vi "Process_Oculus_Data - Rufus.vi"(5 "Arm X Min":dbl, 7 "Arm X Max":dbl, 8 "error in":errorcluster, 9 "Calibration Data in":T3, 10 "Calibrated":bool, 11 "Raw Oculus Data":T1) -> (0 "error out":errorcluster, 1 "Calibration Data out":T3, 3 "Calibrated Oculus Data":T2)   [LabVIEW 2017]
uses:
  Calibrated Oculus Data.ctl
  Raw Oculus Data.ctl
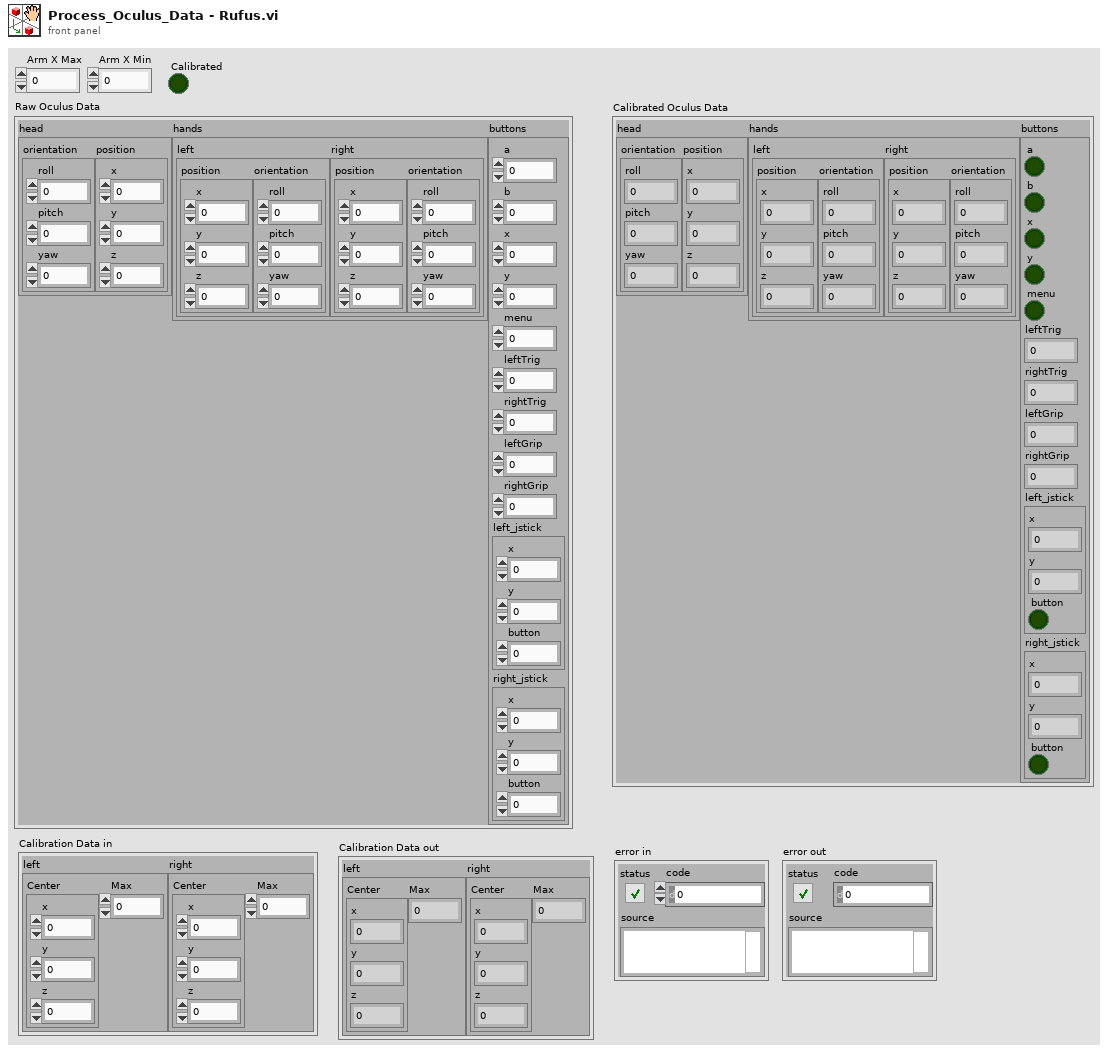
[diagram p1: front panel]
types:
  T1 = typedef "Raw Oculus Data.ctl" = cluster{"head":cluster{"orientation":cluster{"roll":dbl, "pitch":dbl, "yaw":dbl}, "position":cluster{"x":dbl, "y":dbl, "z":dbl}}, "hands":cluster{"left":cluster{"position":cluster{"x":dbl, "y":dbl, "z":dbl}, "orientation":cluster{"roll":dbl, "pitch":dbl, "yaw":dbl}}, "right":cluster{"position":cluster{"x":dbl, "y":dbl, "z":dbl}, "orientation":cluster{"roll":dbl, "pitch":dbl, "yaw":dbl}}}, "buttons":cluster{"a":i32, "b":i32, "x":i32, "y":i32, "menu":i32, "leftTrig":dbl, "rightTrig":dbl, "leftGrip":dbl, "rightGrip":dbl, "left_jstick":cluster{"x":dbl, "y":dbl, "button":i32}, "right_jstick":cluster{"x":dbl, "y":dbl, "button":i32}}}
  T2 = typedef "Calibrated Oculus Data.ctl" = cluster{"head":cluster{"orientation":cluster{"roll":dbl, "pitch":dbl, "yaw":dbl}, "position":cluster{"x":dbl, "y":dbl, "z":dbl}}, "hands":cluster{"left":cluster{"position":cluster{"x":dbl, "y":dbl, "z":dbl}, "orientation":cluster{"roll":dbl, "pitch":dbl, "yaw":dbl}}, "right":cluster{"position":cluster{"x":dbl, "y":dbl, "z":dbl}, "orientation":cluster{"roll":dbl, "pitch":dbl, "yaw":dbl}}}, "buttons":cluster{"a":bool, "b":bool, "x":bool, "y":bool, "menu":bool, "leftTrig":dbl, "rightTrig":dbl, "leftGrip":dbl, "rightGrip":dbl, "left_jstick":cluster{"x":dbl, "y":dbl, "button":bool}, "right_jstick":cluster{"x":dbl, "y":dbl, "button":bool}}}
  T3 = cluster{"left":cluster{"Center":cluster{"x":dbl, "y":dbl, "z":dbl}, "Max":dbl}, "right":cluster{"Center":cluster{"x":dbl, "y":dbl, "z":dbl}, "Max":dbl}}
  T4 = typedef "Calibration Control.ctl" = enum16{"Calibrate", "Max", "Min"}
  T5 = cluster{"orientation":cluster{"roll":dbl, "pitch":dbl, "yaw":dbl}, "position":cluster{"x":dbl, "y":dbl, "z":dbl}}
  T6 = cluster{"left":cluster{"position":cluster{"x":dbl, "y":dbl, "z":dbl}, "orientation":cluster{"roll":dbl, "pitch":dbl, "yaw":dbl}}, "right":cluster{"position":cluster{"x":dbl, "y":dbl, "z":dbl}, "orientation":cluster{"roll":dbl, "pitch":dbl, "yaw":dbl}}}
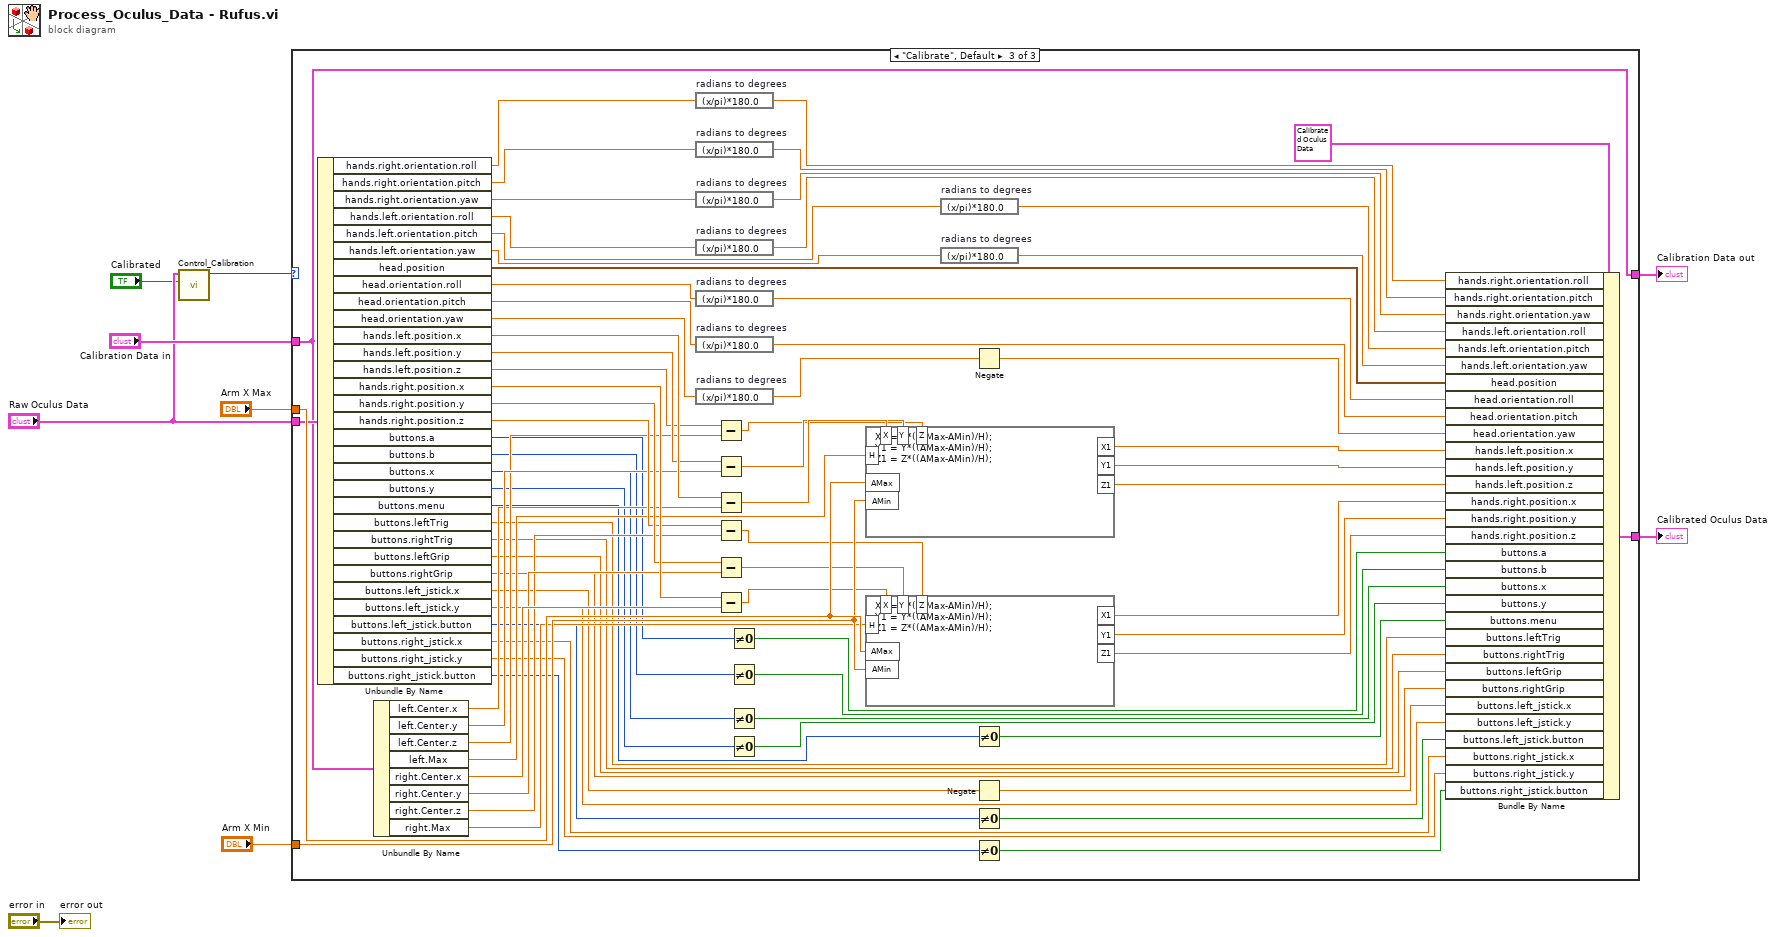
[diagram p0: block diagram]
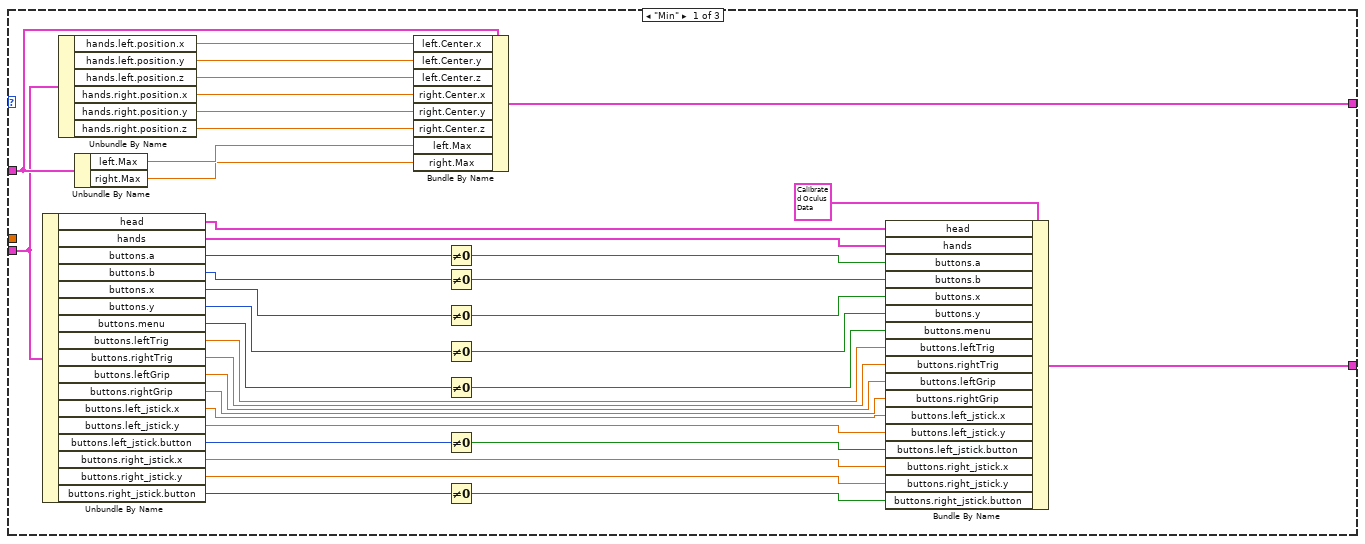
[diagram p2: hidden frame]
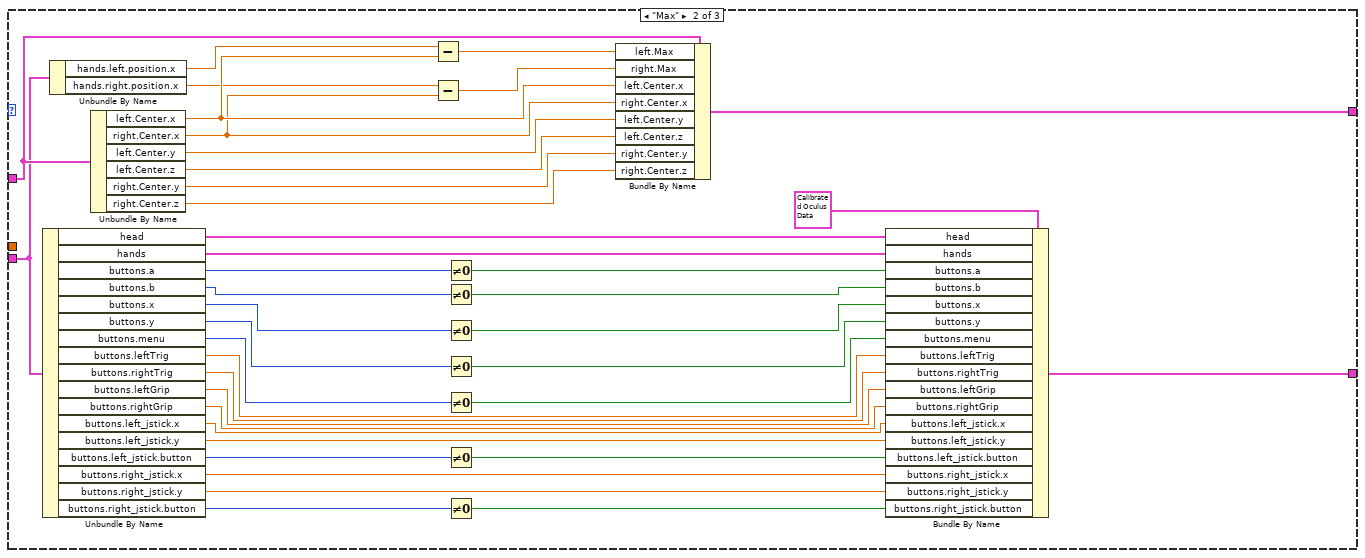
[diagram p3: hidden frame]
diagram:
  n1 = call "Control_Calibration.vi"("Calibrated"="Calibrated", "Raw Oculus Data"="Raw Oculus Data") -> ("Control"=w3:T4)  [unwired: 9 in]
  n2 = case shown="\"Calibrate\", Default" w3 {
    tunnel: "Raw Oculus Data" -> [w12 w73 w149]
    tunnel: "Arm X Max" -> [_ _ w157]
    tunnel: "Arm X Min" -> [_ _ w156]
    tunnel: "Calibration Data in" -> [w46 w76 w135]
    tunnel: [w43 w85 w135] -> w6
    tunnel: [w11 w70 w105] -> w4
    frame "Min" {
      n3 = Unbundle By Name(w12) -> ("head"=w36:T5, "hands"=w35:T6, "buttons.a"=w34:i32, "buttons.b"=w33:i32, "buttons.x"=w32:i32, "buttons.y"=w31:i32, "buttons.menu"=w26:i32, "buttons.leftTrig"=w20:dbl, "buttons.rightTrig"=w19:dbl, "buttons.leftGrip"=w18:dbl, "buttons.rightGrip"=w17:dbl, "buttons.left_jstick.x"=w16:dbl, "buttons.left_jstick.y"=w15:dbl, "buttons.left_jstick.button"=w24:i32, "buttons.right_jstick.x"=w14:dbl, "buttons.right_jstick.y"=w13:dbl, "buttons.right_jstick.button"=w23:i32)
      n4 = Unbundle By Name(w12) -> ("hands.left.position.x"=w42:dbl, "hands.left.position.y"=w41:dbl, "hands.left.position.z"=w40:dbl, "hands.right.position.x"=w39:dbl, "hands.right.position.y"=w38:dbl, "hands.right.position.z"=w37:dbl)
      n5 = Unbundle By Name(w46) -> ("left.Max"=w45:dbl, "right.Max"=w44:dbl)
      n6 = Bundle By Name(cluster=w46, "left.Center.x"=w42, "left.Center.y"=w41, "left.Center.z"=w40, "right.Center.x"=w39, "right.Center.y"=w38, "right.Center.z"=w37, "left.Max"=w45, "right.Max"=w44) -> (w43:T3)
      n7 = Not Equal To 0?(x=w34) -> (x != 0?=w30:bool)
      n8 = Not Equal To 0?(x=w33) -> (x != 0?=w29:bool)
      n9 = Not Equal To 0?(x=w32) -> (x != 0?=w28:bool)
      n10 = Not Equal To 0?(x=w31) -> (x != 0?=w27:bool)
      n11 = Not Equal To 0?(x=w26) -> (x != 0?=w25:bool)
      n12 = Not Equal To 0?(x=w24) -> (x != 0?=w22:bool)
      n13 = Not Equal To 0?(x=w23) -> (x != 0?=w21:bool)
      n14 = Bundle By Name(cluster=T2 {"head"={"orientation"={"roll"=0.0, "pitch"=0.0, "yaw"=0.0}, "position"={"x"=0.0, "y"=0.0, "z"=0.0}}, "hands"={"left"={"position"={"x"=0.0, "y"=0.0, "z"=0.0}, "orientation"={"roll"=0.0, "pitch"=0.0, "yaw"=0.0}}, "right"={"position"={"x"=0.0, "y"=0.0, "z"=0.0}, "orientation"={"roll"=0.0, "pitch"=0.0, "yaw"=0.0}}}, "buttons"={"a"=FALSE, "b"=FALSE, "x"=FALSE, "y"=FALSE, "menu"=FALSE, "leftTrig"=0.0, "rightTrig"=0.0, "leftGrip"=0.0, "rightGrip"=0.0, "left_jstick"={"x"=0.0, "y"=0.0, "button"=FALSE}, "right_jstick"={"x"=0.0, "y"=0.0, "button"=FALSE}}} ("Calibrated Oculus Data"), "head"=w36, "hands"=w35, "buttons.a"=w30, "buttons.b"=w29, "buttons.x"=w28, "buttons.y"=w27, "buttons.menu"=w25, "buttons.leftTrig"=w20, "buttons.rightTrig"=w19, "buttons.leftGrip"=w18, "buttons.rightGrip"=w17, "buttons.left_jstick.x"=w16, "buttons.left_jstick.y"=w15, "buttons.left_jstick.button"=w22, "buttons.right_jstick.x"=w14, "buttons.right_jstick.y"=w13, "buttons.right_jstick.button"=w21) -> (w11:T2)
    }
    frame "Max" {
      n15 = Unbundle By Name(w73) -> ("head"=w72:T5, "hands"=w71:T6, "buttons.a"=w69:i32, "buttons.b"=w68:i32, "buttons.x"=w67:i32, "buttons.y"=w66:i32, "buttons.menu"=w61:i32, "buttons.leftTrig"=w55:dbl, "buttons.rightTrig"=w54:dbl, "buttons.leftGrip"=w53:dbl, "buttons.rightGrip"=w52:dbl, "buttons.left_jstick.x"=w51:dbl, "buttons.left_jstick.y"=w50:dbl, "buttons.left_jstick.button"=w59:i32, "buttons.right_jstick.x"=w49:dbl, "buttons.right_jstick.y"=w48:dbl, "buttons.right_jstick.button"=w58:i32)
      n16 = Unbundle By Name(w73) -> ("hands.left.position.x"=w75:dbl, "hands.right.position.x"=w74:dbl)
      n17 = Unbundle By Name(w76) -> ("left.Center.x"=w84:dbl, "right.Center.x"=w83:dbl, "left.Center.y"=w82:dbl, "left.Center.z"=w81:dbl, "right.Center.y"=w80:dbl, "right.Center.z"=w79:dbl)
      n18 = Subtract(x=w75, y=w84) -> (x-y=w78:dbl)
      n19 = Subtract(x=w74, y=w83) -> (x-y=w77:dbl)
      n20 = Not Equal To 0?(x=w69) -> (x != 0?=w65:bool)
      n21 = Not Equal To 0?(x=w68) -> (x != 0?=w64:bool)
      n22 = Not Equal To 0?(x=w67) -> (x != 0?=w63:bool)
      n23 = Not Equal To 0?(x=w66) -> (x != 0?=w62:bool)
      n24 = Not Equal To 0?(x=w61) -> (x != 0?=w60:bool)
      n25 = Not Equal To 0?(x=w59) -> (x != 0?=w57:bool)
      n26 = Not Equal To 0?(x=w58) -> (x != 0?=w56:bool)
      n27 = Bundle By Name(cluster=w76, "left.Max"=w78, "right.Max"=w77, "left.Center.x"=w84, "right.Center.x"=w83, "left.Center.y"=w82, "left.Center.z"=w81, "right.Center.y"=w80, "right.Center.z"=w79) -> (w85:T3)
      n28 = Bundle By Name(cluster=T2 {"head"={"orientation"={"roll"=0.0, "pitch"=0.0, "yaw"=0.0}, "position"={"x"=0.0, "y"=0.0, "z"=0.0}}, "hands"={"left"={"position"={"x"=0.0, "y"=0.0, "z"=0.0}, "orientation"={"roll"=0.0, "pitch"=0.0, "yaw"=0.0}}, "right"={"position"={"x"=0.0, "y"=0.0, "z"=0.0}, "orientation"={"roll"=0.0, "pitch"=0.0, "yaw"=0.0}}}, "buttons"={"a"=FALSE, "b"=FALSE, "x"=FALSE, "y"=FALSE, "menu"=FALSE, "leftTrig"=0.0, "rightTrig"=0.0, "leftGrip"=0.0, "rightGrip"=0.0, "left_jstick"={"x"=0.0, "y"=0.0, "button"=FALSE}, "right_jstick"={"x"=0.0, "y"=0.0, "button"=FALSE}}} ("Calibrated Oculus Data"), "head"=w72, "hands"=w71, "buttons.a"=w65, "buttons.b"=w64, "buttons.x"=w63, "buttons.y"=w62, "buttons.menu"=w60, "buttons.leftTrig"=w55, "buttons.rightTrig"=w54, "buttons.leftGrip"=w53, "buttons.rightGrip"=w52, "buttons.left_jstick.x"=w51, "buttons.left_jstick.y"=w50, "buttons.left_jstick.button"=w57, "buttons.right_jstick.x"=w49, "buttons.right_jstick.y"=w48, "buttons.right_jstick.button"=w56) -> (w70:T2)
    }
    frame "Calibrate", Default {
      n29 = Unbundle By Name(w149) -> ("hands.right.orientation.roll"=w116:dbl, "hands.right.orientation.pitch"=w115:dbl, "hands.right.orientation.yaw"=w114:dbl, "hands.left.orientation.roll"=w110:dbl, "hands.left.orientation.pitch"=w109:dbl, "hands.left.orientation.yaw"=w108:dbl, "head.position"=w148:cluster{"x":dbl, "y":dbl, "z":dbl}, "head.orientation.roll"=w152:dbl, "head.orientation.pitch"=w151:dbl, "head.orientation.yaw"=w150:dbl, "hands.left.position.x"=w144:dbl, "hands.left.position.y"=w143:dbl, "hands.left.position.z"=w142:dbl, "hands.right.position.x"=w141:dbl, "hands.right.position.y"=w140:dbl, "hands.right.position.z"=w139:dbl, "buttons.a"=w126:i32, "buttons.b"=w120:i32, "buttons.x"=w124:i32, "buttons.y"=w121:i32, "buttons.menu"=w104:i32, "buttons.leftTrig"=w118:dbl, "buttons.rightTrig"=w117:dbl, "buttons.leftGrip"=w94:dbl, "buttons.rightGrip"=w93:dbl, "buttons.left_jstick.x"=w102:dbl, "buttons.left_jstick.y"=w101:dbl, "buttons.left_jstick.button"=w100:i32, "buttons.right_jstick.x"=w98:dbl, "buttons.right_jstick.y"=w97:dbl, "buttons.right_jstick.button"=w96:i32)
      n30 = Unbundle By Name(w135) -> ("left.Center.x"=w132:dbl, "left.Center.y"=w134:dbl, "left.Center.z"=w133:dbl, "left.Max"=w131:dbl, "right.Center.x"=w130:dbl, "right.Center.y"=w129:dbl, "right.Center.z"=w128:dbl, "right.Max"=w127:dbl)
      n31 = expression code="(x/pi)*180.0" "radians to degrees"(w116) -> (w113:dbl)
      n32 = expression code="(x/pi)*180.0" "radians to degrees"(w115) -> (w112:dbl)
      n33 = expression code="(x/pi)*180.0" "radians to degrees"(w114) -> (w111:dbl)
      n34 = expression code="(x/pi)*180.0" "radians to degrees"(w110) -> (w107:dbl)
      n35 = expression code="(x/pi)*180.0" "radians to degrees"(w152) -> (w90:dbl)
      n36 = expression code="(x/pi)*180.0" "radians to degrees"(w151) -> (w89:dbl)
      n37 = expression code="(x/pi)*180.0" "radians to degrees"(w150) -> (w88:dbl)
      n38 = Subtract(x=w142, y=w133) -> (x-y=w158:dbl)
      n39 = Subtract(x=w143, y=w134) -> (x-y=w159:dbl)
      n40 = Subtract(x=w144, y=w132) -> (x-y=w160:dbl)
      n41 = Subtract(x=w139, y=w128) -> (x-y=w153:dbl)
      n42 = Subtract(x=w140, y=w129) -> (x-y=w154:dbl)
      n43 = Subtract(x=w141, y=w130) -> (x-y=w155:dbl)
      n44 = Not Equal To 0?(x=w126) -> (x != 0?=w125:bool)
      n45 = Not Equal To 0?(x=w120) -> (x != 0?=w119:bool)
      n46 = Not Equal To 0?(x=w124) -> (x != 0?=w123:bool)
      n47 = Not Equal To 0?(x=w121) -> (x != 0?=w122:bool)
      n48 = formula code="X1 = X*((AMax-AMin)/H);\nY1 = Y*((AMax-AMin)/H);\nZ1 = Z*((AMax-AMin)/H);"("H"=w131, "AMax"=w157, "X"=w160, "Y"=w159, "Z"=w158, "AMin"=w156) -> ("X1"=w147:dbl, "Y1"=w146:dbl, "Z1"=w145:dbl)
      n49 = formula code="X1 = X*((AMax-AMin)/H);\nY1 = Y*((AMax-AMin)/H);\nZ1 = Z*((AMax-AMin)/H);"("H"=w127, "AMax"=w157, "X"=w155, "Y"=w154, "Z"=w153, "AMin"=w156) -> ("X1"=w138:dbl, "Y1"=w137:dbl, "Z1"=w136:dbl)
      n50 = expression code="(x/pi)*180.0" "radians to degrees"(w109) -> (w91:dbl)
      n51 = expression code="(x/pi)*180.0" "radians to degrees"(w108) -> (w106:dbl)
      n52 = Negate(x=w88) -> (-x=w87:dbl)
      n53 = Not Equal To 0?(x=w104) -> (x != 0?=w103:bool)
      n54 = Negate(x=w102) -> (-x=w86:dbl)
      n55 = Not Equal To 0?(x=w100) -> (x != 0?=w99:bool)
      n56 = Not Equal To 0?(x=w96) -> (x != 0?=w95:bool)
      n57 = Bundle By Name(cluster=T2 {"head"={"orientation"={"roll"=0.0, "pitch"=0.0, "yaw"=0.0}, "position"={"x"=0.0, "y"=0.0, "z"=0.0}}, "hands"={"left"={"position"={"x"=0.0, "y"=0.0, "z"=0.0}, "orientation"={"roll"=0.0, "pitch"=0.0, "yaw"=0.0}}, "right"={"position"={"x"=0.0, "y"=0.0, "z"=0.0}, "orientation"={"roll"=0.0, "pitch"=0.0, "yaw"=0.0}}}, "buttons"={"a"=FALSE, "b"=FALSE, "x"=FALSE, "y"=FALSE, "menu"=FALSE, "leftTrig"=0.0, "rightTrig"=0.0, "leftGrip"=0.0, "rightGrip"=0.0, "left_jstick"={"x"=0.0, "y"=0.0, "button"=FALSE}, "right_jstick"={"x"=0.0, "y"=0.0, "button"=FALSE}}} ("Calibrated Oculus Data"), "hands.right.orientation.roll"=w113, "hands.right.orientation.pitch"=w112, "hands.right.orientation.yaw"=w111, "hands.left.orientation.roll"=w107, "hands.left.orientation.pitch"=w91, "hands.left.orientation.yaw"=w106, "head.position"=w148, "head.orientation.roll"=w90, "head.orientation.pitch"=w89, "head.orientation.yaw"=w87, "hands.left.position.x"=w147, "hands.left.position.y"=w146, "hands.left.position.z"=w145, "hands.right.position.x"=w138, "hands.right.position.y"=w137, "hands.right.position.z"=w136, "buttons.a"=w125, "buttons.b"=w119, "buttons.x"=w123, "buttons.y"=w122, "buttons.menu"=w103, "buttons.leftTrig"=w118, "buttons.rightTrig"=w117, "buttons.leftGrip"=w94, "buttons.rightGrip"=w93, "buttons.left_jstick.x"=w86, "buttons.left_jstick.y"=w101, "buttons.left_jstick.button"=w99, "buttons.right_jstick.x"=w98, "buttons.right_jstick.y"=w97, "buttons.right_jstick.button"=w95) -> (w105:T2)
    }
  }
  "Calibration Data out" <- w6
  "Calibrated Oculus Data" <- w4
  "error out" <- "error in"
